vi "Add Rx Frames.vi"(8 "error in (no error)":errorcluster, 10 "Frames":variant, 11 "LINBus_Load_Calculator in":refnum<class "LINBus_Load_Calculator.lvclass">) -> (0 "error out":errorcluster, 3 "LINBus_Load_Calculator out":refnum<class "LINBus_Load_Calculator.lvclass">)   [LabVIEW 2019, in "XNET-Bus-Load-Calculator.lvlib" / "LINBus_Load_Calculator.lvclass"]
uses:
  LINBus_Load_Calculator.lvclass
  GenBus/GenBus_Load_Calculator.lvclass
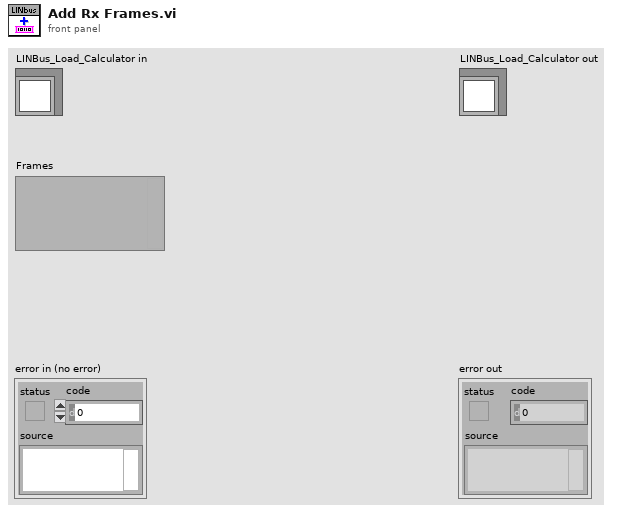
[diagram p1: front panel]
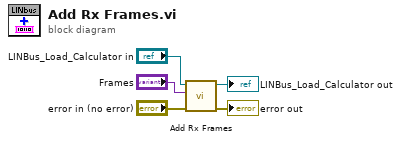
[diagram p0: block diagram]
diagram:
  n1 = call-parent "Add Rx Frames.vi"("error in (no error)"="error in (no error)", "Frames"="Frames", "GenBus_Load_Calculator in"="LINBus_Load_Calculator in") -> ("error out"=→"error out":errorcluster, "GenBus_Load_Calculator out"=→"LINBus_Load_Calculator out":refnum<class "LINBus_Load_Calculator.lvclass">)  [unwired: 7 in]
